vi "Acquire N Scans Analog Software Trig V1.vi"(0 "device":i16=1, 1 "trigger channel":string="0", 2 "time limit (sec)":sgl=5.0 format="%.2f", 7 "number of scans\nto acquire":i32=1000, 9 "scan rate":sgl=1000.0 format="%.2f", 11 "input limits":cluster{"high limit":sgl, "low limit":sgl}[](array[cluster])=[{"high limit"=1.0, "low limit"=-1.0}] {"low limit" format="%.2f"; "high limit" format="%.2f"}, 12 "pretrigger scans":i32, 13 "trigger slope":enum16{"no change", "rising", "falling"}(ring)=enum."rising", 14 "trigger level":sgl format="%.2f") -> (4 "data":waveform(dbl)[](array[waveform]), 6 "timeout?":bool)   [LabVIEW 2022 SP3]
doc: "DESCRIPTION:\nThis VI retrieves the specified amount of data from one or more analog input channels when a software analog trigger occurs. This is a timed acquisition, meaning that a hardware clock is used to control the acquisition rate for fast and accurate timing. It is also a buffered acquisition, meaning that the data are stored in an intermediate memory buffer after they are acquired from the DAQ board. Since this VI uses a software analog trigger, data are continuously acquired with LabVIEW checking the intermediate buffer for the analog trigger specifications to be met. Once met, this VI retrieves and displays data from that buffer after the appropriate amount of data (before and after the trigger) have been acquired. The vertical cursor on the graph indicates where the trigger occurred.\n\nUse this VI to wait for a software analog trigger, acquiring a relatively small amount of data (it must fit in the memory available), where each point does not need to be viewed or processed while it is being acquired\n\nINSTRUCTIONS:\n1. Enter the device number, channels, trigger channel, number of scans to acquire, and the scan rate.\n2. Enter the pretrigger scans, trigger slope, trigger level, and time limit.\n3. Make the appropriate I/O connections as explained below.\n4. Run the VI.\n\nKEY PARAMETERS:\nThis VI shows how to use the intermediate analog input DAQ VIs to software trigger an acquisition.\n\nCalculate Buffer Size.vi is used to allocate a buffer which is the largest of the following: 1000 scans, 400 msec worth of scans, or 2.5 times the \"number of scans to acquire\". This tries to provide enough cushion for the driver to keep up in searching for the trigger condition while data are acquired. It is still possible for the VI to overflow the buffer or time-out if the acquisition speed is high.\n\nSet up Conditional Retrieval.vi provides trigger parameters, the trigger channel index, and turns on conditional retrieval in AI Read.vi.\n\nThe \"read/search mode\" for AI Read.vi is set to \"relative to end of data\". This assures that LabVIEW checks the most recently acquired data (end of data) for the software trigger.\n\nI/O CONNECTIONS:\nConnect to the input channels on the I/O connector for your board to match the channels you have chosen on the front panel of this VI. For example ACH0 for analog input.\n\nTo find the actual pin numbers, refer to your hardware user manual.\n\nDAQ VIs USED:\nAI Config.vi, AI Start.vi, AI Read.vi, AI Clear.vi."
uses:
  Doppler/dopplerV6.llb/AI Read (waveform).vi
panel:
  in  "channels":tag[](array[tag])=["I", "Q"]
  out "waveform graph":waveform(dbl)[](graph)
  in  "hysteresis":sgl=0.1 format="%.2f"
  # "For instructions select File >> VI Properties >> Documentation"
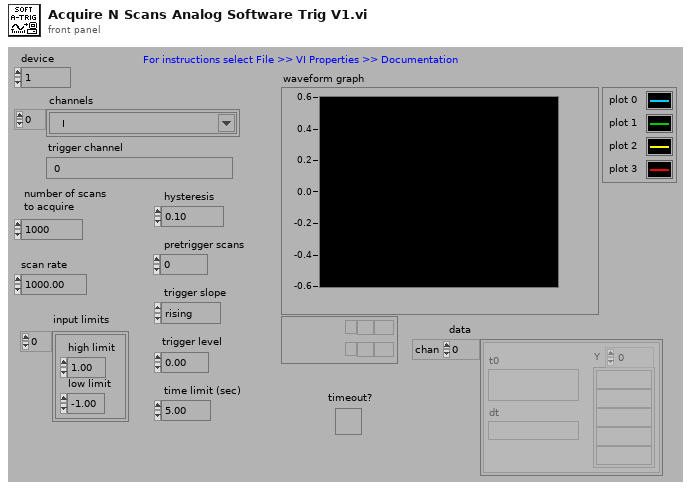
[diagram p1: front panel]
types:
  T1 = enum16{"no change", "relative to read mark", "relative to start of buffer", "relative to end of data", "relative to trigger point"}
  T2 = cluster{"trigger channel":string, "trigger level":sgl}
  T3 = cluster{"read/search mode":enum16{"no change", "relative to read mark", "relative to start of buffer", "relative to end of data", "relative to trigger point"}, "read offset":i32}
  T4 = cluster{"mode (off)":enum16{"no change", "off", "on"}, "channel index (0)":i32, "slope (rising)":enum16{"no change", "rising", "falling"}, "level (0.0)":sgl, "hysteresis (0.0)":sgl, "skip count (0)":i32, "offset (0)":i32}
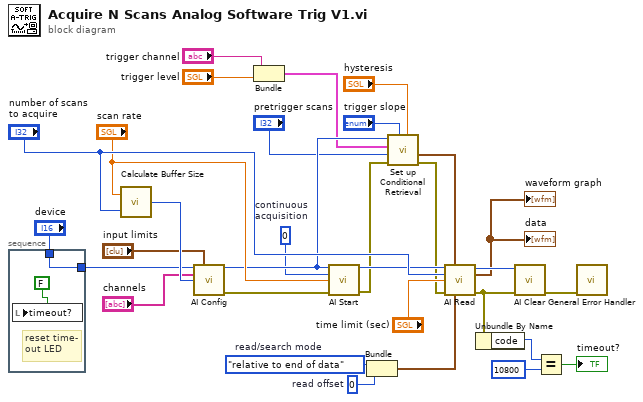
[diagram p0: block diagram]
diagram:
  w4 = 0  # continuous acquisition
  w21 = T1."relative to end of data"  # read/search mode
  w22 = 0  # read offset
  n1 = stacked-sequence {
    tunnel: [w32] -> w16
    tunnel: "device" -> [w32]
    frame #0 {
      # "reset time-\nout LED"
      n2 = local write "timeout?"(FALSE) -> ()
    }
  }
  n3 = call "Calculate Buffer Size.vi"("number of scans\nto acquire"="number of scans\nto acquire", "scan rate"="scan rate") -> ("buffer size"=w17:i32)
  n4 = call "AI Config.vi"("device (1)"=w16, "input limits (no change)"="input limits", "channels (0)"="channels", "buffer size (1000 scans)"=w17) -> ("taskID"=w11:u32, "error out"=w19:errorcluster)  [unwired: 9 in, 1 out]
  n5 = Bundle("trigger channel"="trigger channel", "trigger level"="trigger level") -> (w7:T2)  [unwired: 1 in]
  n6 = call "AI Start.vi"("taskID in"=w11, "number of scans to acquire (-1)"=w4, "scan rate (1000 scans/sec)"="scan rate", "error in (no error)"=w19) -> ("taskID out"=w18:u32, "error out"=w10:errorcluster)  [unwired: 8 in, 2 out]
  n7 = Bundle("read/search mode"=w21, "read offset"=w22) -> (w26:T3)  [unwired: 1 in]
  n8 = call "Set up Conditional Retrieval.vi"("hysteresis (1 V)"="hysteresis", "trig slope (rising)"="trigger slope", "error in"=w10, "pretrigger\nscans (0)"="pretrigger scans", "analog chan (-) & level (0)"=w7, "taskID"=w11) -> ("error out"=w9:errorcluster, "conditional retrieval"=w6:T4)  [unwired: 3 in, 1 out]
  n9 = call-poly "AI Read.vi"("taskID in"=w18, "conditional retrieval (off)"=w6, "number of scans to read (-1:all)"="number of scans\nto acquire", "time limit in sec (-1:auto calculate)"="time limit (sec)", "error in (no error)"=w9, "read/search position (from mark)"=w26) -> ("taskID out"=w13:u32, "waveform data"=→"waveform graph" →"data":waveform(dbl)[], "error out"=w14:errorcluster)  [unwired: 4 in, 3 out]
  n10 = Unbundle By Name(w14) -> ("code"=w25:i32)
  n11 = call "AI Clear.vi"("error in (no error)"=w14, "taskID in"=w13) -> ("error out"=w31:errorcluster)  [unwired: 4 in, 1 out]
  n12 = Equal?(x=w25, y=10800) -> (x = y?=→"timeout?":bool)
  n13 = call <vilib>:"General Error Handler.vi"("error in (no error)"=w31) -> ()  [unwired: 10 in, 5 out]
